vi "Serial Port Lister.vi"() -> ()   [LabVIEW 2021]
doc: "VI to show all serial ports and their system name.\nScott Hannahs sth@infolabview.org"
panel:
  out "Cycle Time":dbl format="%.3f"
  out "Port":string[](array[string])
  out "Valid":bool[](array[boolean])
  out "return count":i32
  out "VISA Name":string[](array[string])
  in  "stop":bool
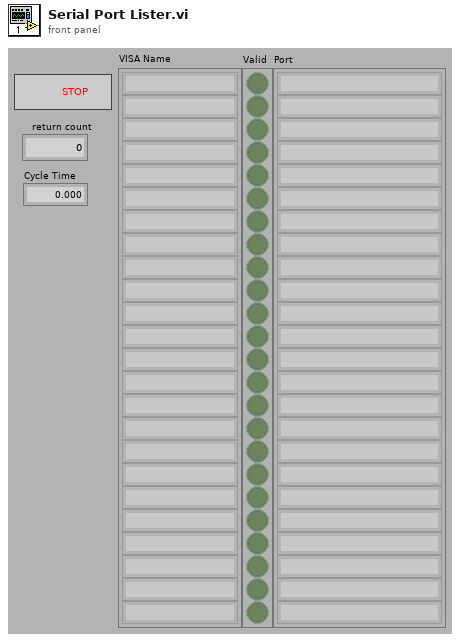
[diagram p1: front panel]
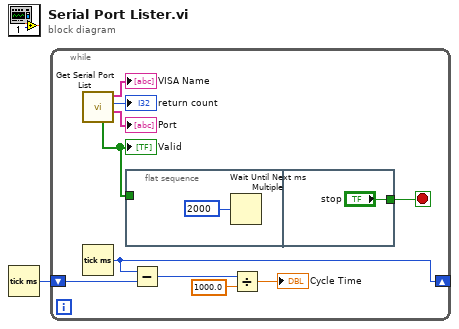
[diagram p0: block diagram]
diagram:
  n1 = Tick Count (ms)() -> (millisecond timer value=w1:u32)
  n2 = while {
    shift-right: [w6] -> _
    shift-left: w1 -> [w2]
    stop <- w11 stop-if-true
    n3 = call "Get Serial Port List.vi"() -> ("Port Names"=→"Port":string[], "#Ports"=→"return count":i32, "VISA Name"=→"VISA Name":string[], "Valid"=w8:bool[])  [unwired: 7 in, 1 out]
    "Valid" <- w8
    n4 = Tick Count (ms)() -> (millisecond timer value=w6:u32)
    n5 = flat-sequence {
      tunnel: w8 -> [_]
      tunnel: ["stop"] -> w11
      frame #0 {
        n6 = Wait Until Next ms Multiple(millisecond multiple=u32 2000) -> ()  [unwired: 1 out]
      }
      frame #1 {
      }
    }
    n7 = Subtract(x=w6, y=w2) -> (x-y=w5:u32)
    n8 = Divide(x=w5, y=1000.0) -> (x/y=→"Cycle Time":dbl)
  }
